vi "Desktop Main.vi"() -> ()   [LabVIEW 2021]
doc: "Demonstrates how to use a generator and message queues to send data to the myRIO target."
panel:
  in  "Target Port":u16=58432
  in  "Stop":bool
  in  "Message Queue":string="Desktop"
  in  "Target IP Address":string="172.22.11.2"
  in  "Target Queue Name":string="Target"
  out "Tank":dbl(slide) scale=0.0..10.0
  out "error out":errorcluster
  in  "Local Port":u16=58431
  # "Overview: Demonstrates how to use a generator and message queues to send data to the myRIO target.\nInstructions:\n1. Run this VI.\n2. Open RT Main.vi and follow its front panel instructions.\n3. Click Stop to stop this VI."
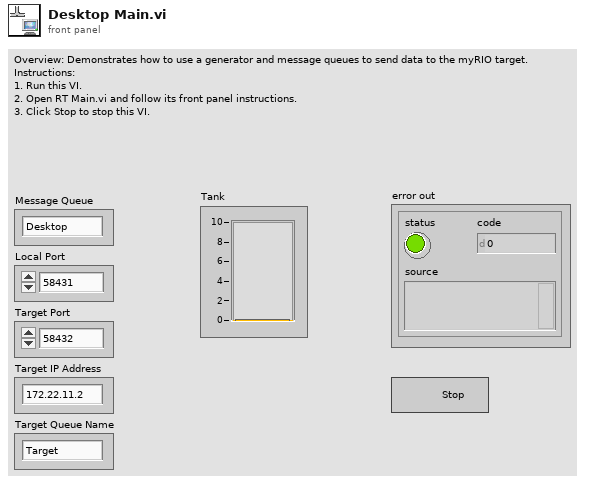
[diagram p1: front panel]
types:
  T1 = typedef "Message.ctl" = cluster{"Name":string, "Value":string, "Local IP":string, "Local Queue":string, "Remote IP":string, "Remote Queue":string}
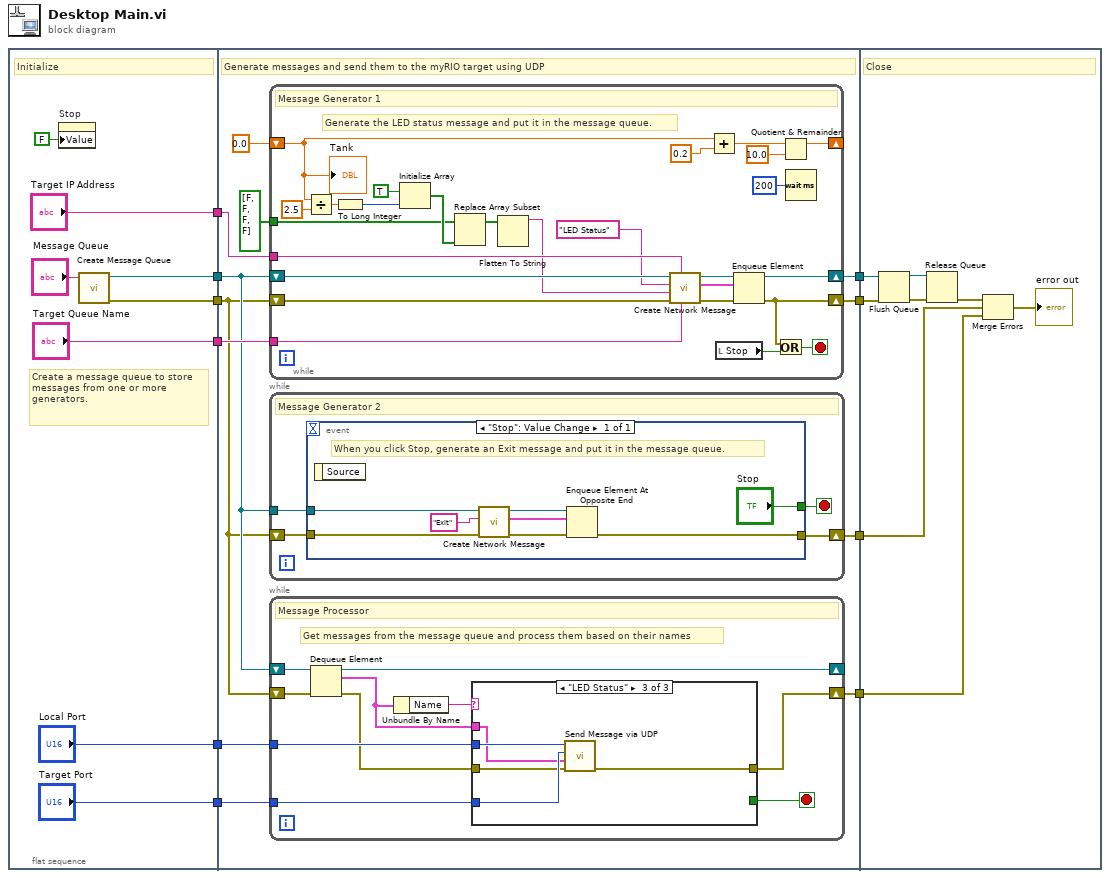
[diagram p0: block diagram]
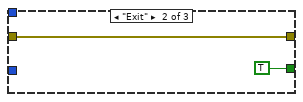
[diagram p3: hidden frame]
diagram:
  n1 = flat-sequence {
    tunnel: [w18] -> w10
    tunnel: [w17] -> w9
    tunnel: ["Target IP Address"] -> w8
    tunnel: ["Target Queue Name"] -> w7
    tunnel: ["Local Port"] -> w6
    tunnel: ["Target Port"] -> w5
    tunnel: w10 -> [w27]
    tunnel: w9 -> [w21]
    tunnel: w8 -> [w29]
    tunnel: w7 -> [w28]
    tunnel: w6 -> [w26]
    tunnel: w5 -> [w25]
    tunnel: [w24] -> w4
    tunnel: [w23] -> w3
    tunnel: [w22] -> w2
    tunnel: [w20] -> w1
    tunnel: w4 -> [w90]
    tunnel: w3 -> [w89]
    tunnel: w2 -> [w86]
    tunnel: w1 -> [w85]
    frame #0 {
      # "Create a message queue to store messages from one or more generators."
      # "Initialize"
      n2 = property on="Stop" class="Bool (strict)"("Value"=FALSE ("Stop")) -> ()  [unwired: 2 in, 2 out]
      n3 = call "Create Message Queue.vi"("queue name"="Message Queue") -> ("error out"=w17:errorcluster, "Message queue"=w18:refnum<queue>)  [unwired: 9 in]
    }
    frame #1 {
      # "Generate messages and send them to the myRIO target using UDP"
      n4 = while {
        shift-right: [w76] -> _
        shift-left: 0.0 -> [w80]
        shift-right: [w71] -> w24
        shift-left: w27 -> [w73]
        shift-right: [w66] -> w23
        shift-left: w21 -> [w70]
        tunnel: w29 -> [w74]
        tunnel: w28 -> [w75]
        tunnel: bool[] [FALSE, FALSE, FALSE, FALSE] -> [w61]
        stop <- w84 stop-if-true
        # "Generate the LED status message and put it in the message queue."
        # "Message Generator 1"
        n5 = Divide(x=w80, y=2.5) -> (x/y=w82:dbl)
        n6 = To Long Integer(number=w82) -> (32bit integer=w64:i32)
        n7 = Initialize Array(TRUE, w64) -> (w63:bool[])
        n8 = Replace Array Subset(array=w61, new element=w63) -> (w62:bool[])  [unwired: 1 in]
        n9 = Flatten To String(anything=w62) -> (data string=w68:string)  [unwired: 3 in, 2 out]
        n10 = call "Create Network Message.vi"("Remote Process"=w75, "Remote IP"=w74, "Value"=w68, "Name"="LED Status", "Message queue"=w73) -> ("Message"=w69:T1, "Message queue out"=w72:refnum<queue>)  [unwired: 5 in]
        n11 = Add(x=w80, y=0.2) -> (x+y=w77:dbl)
        n12 = local read "Stop"() -> (w60:bool)
        n13 = Enqueue Element(queue=w72, element=w69, error in (no error)=w70) -> (queue out=w71:refnum<queue>, error out=w66:errorcluster)  [unwired: 1 in, 1 out]
        n14 = Or(x=w66, y=w60) -> (x .or. y?=w84:bool)
        n15 = Quotient & Remainder(x=w77, y=10.0) -> (x-y*floor(x/y)=w76:dbl)  [unwired: 1 out]
        n16 = Wait (ms)(milliseconds to wait=u32 200) -> ()  [unwired: 1 out]
        "Tank" <- w80
      }
      n17 = while {
        tunnel: w27 -> [w51]
        shift-right: [w49] -> w20
        shift-left: w21 -> [w50]
        stop <- w52 stop-if-true
        # "Message Generator 2"
        n18 = event shown="[0] \"Stop\": Value Change" {
          selector: _ -> [_]
          dyn-events: _ -> [_]
          timeout: _ -> [_]
          tunnel: ["Stop"] -> w52
          tunnel: w51 -> [w58]
          tunnel: w50 -> [w54]
          tunnel: [w53] -> w49
          event "Stop": Value Change {
            # "When you click Stop, generate an Exit message and put it in the message queue."
            n19 = event-data() -> ()  [unwired: 1 in, 1 out]
            n20 = call "Create Network Message.vi"("Name"="Exit", "Message queue"=w58) -> ("Message"=w55:T1, "Message queue out"=w56:refnum<queue>)  [unwired: 8 in]
            n21 = Enqueue Element At Opposite End(queue=w56, element=w55, error in (no error)=w54) -> (error out=w53:errorcluster)  [unwired: 1 in, 2 out]
          }
        }
      }
      n22 = while {
        shift-right: [w33] -> _
        shift-left: w27 -> [w40]
        tunnel: w26 -> [w37]
        tunnel: w25 -> [w36]
        shift-right: [w31] -> w22
        shift-left: w21 -> [w39]
        stop <- w32 stop-if-true
        # "Get messages from the message queue and process them based on their names"
        # "Message Processor"
        n23 = Dequeue Element(queue=w40, error in (no error)=w39) -> (queue out=w33:refnum<queue>, element=w35:T1, error out=w34:errorcluster)  [unwired: 1 in, 1 out]
        n24 = Unbundle By Name(w35) -> ("Name"=w38:string)
        n25 = case shown="\"LED Status\"" w38 {
          tunnel: w37 -> [_ _ w48]
          tunnel: w36 -> [_ _ w47]
          tunnel: w35 -> [_ _ w46]
          tunnel: w34 -> [w41 w43 w45]
          tunnel: [w41 w43 w44] -> w31
          tunnel: [_ TRUE _] -> w32
          frame Default {
          }
          frame "Exit" {
          }
          frame "LED Status" {
            n26 = call "Send Message via UDP.vi"("error in"=w45, "Message"=w46, "Remote Port"=w47, "Local Port"=w48) -> ("error out"=w44:errorcluster)  [unwired: 7 in]
          }
        }
      }
    }
    frame #2 {
      # "Close"
      n27 = Flush Queue(queue=w90, error in (no error)=w89) -> (queue out=w91:refnum<queue>, error out=w92:errorcluster)  [unwired: 1 out]
      n28 = Release Queue(queue=w91, error in (no error)=w92) -> (error out=w88:errorcluster)  [unwired: 1 in, 2 out]
      n29 = Merge Errors(w88, w85, w86) -> (→"error out":errorcluster)
    }
  }
